vi "New JSON (Null).vi"(8 "error in (no error)":errorcluster) -> (0 "error out":errorcluster, 3 "JSON Value out":refnum<class "JSON Value.lvclass">)   [LabVIEW 2016, in "JSON Value.lvclass"]
doc: "Create a new JSON instance with no assigned value"
uses:
  JSON Value.lvclass
  JSON Types.ctl
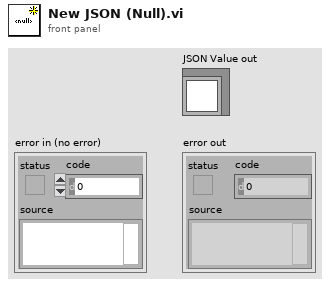
[diagram p1: front panel]
types:
  T1 = typedef "JSON Value.lvclass/JSON Types.ctl" = enum16{"String", "Numeric", "Boolean", "NULL", "Object", "Array"}
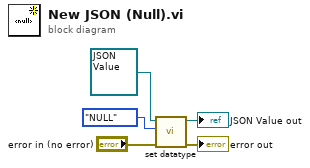
[diagram p0: block diagram]
diagram:
  n1 = call "set datatype.vi"("error in (no error)"="error in (no error)", "datatype"=JSON_Types."NULL", "JSON Helper in"=refnum<class "JSON Value.lvclass"> refnum ("JSON out")) -> ("error out"=→"error out":errorcluster, "JSON Helper out"=→"JSON Value out":refnum<class "JSON Value.lvclass">)  [unwired: 7 in]
